vi "MTS_AutoZPos.vi"(0 "PH Dev":i32, 1 "OFlow Interv [s]":dbl, 2 "Accum Time [s]":dbl=0.1, 5 "PI System no.":i32, 11 "error in":errorcluster, 12 "Start Point":T1, 13 "Steps":i32=9, 14 "Step Width [um]":dbl=0.5) -> (4 "New Z":dbl, 6 "Counts":u32[](array[numeric]), 8 "Position":dbl[](array[numeric]), 15 "error out":errorcluster)   [LabVIEW 2013]
panel:
  out "FiFo Overrun":bool
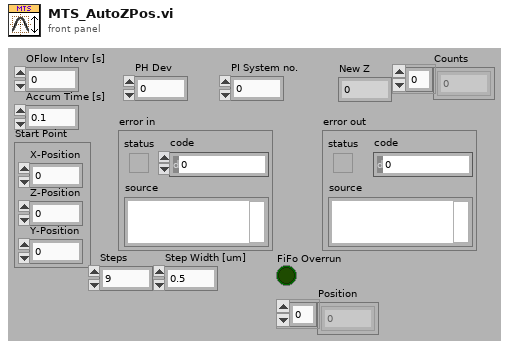
[diagram p1: front panel]
types:
  T1 = cluster{"X-Position":dbl, "Y-Position":dbl, "Z-Position":dbl}
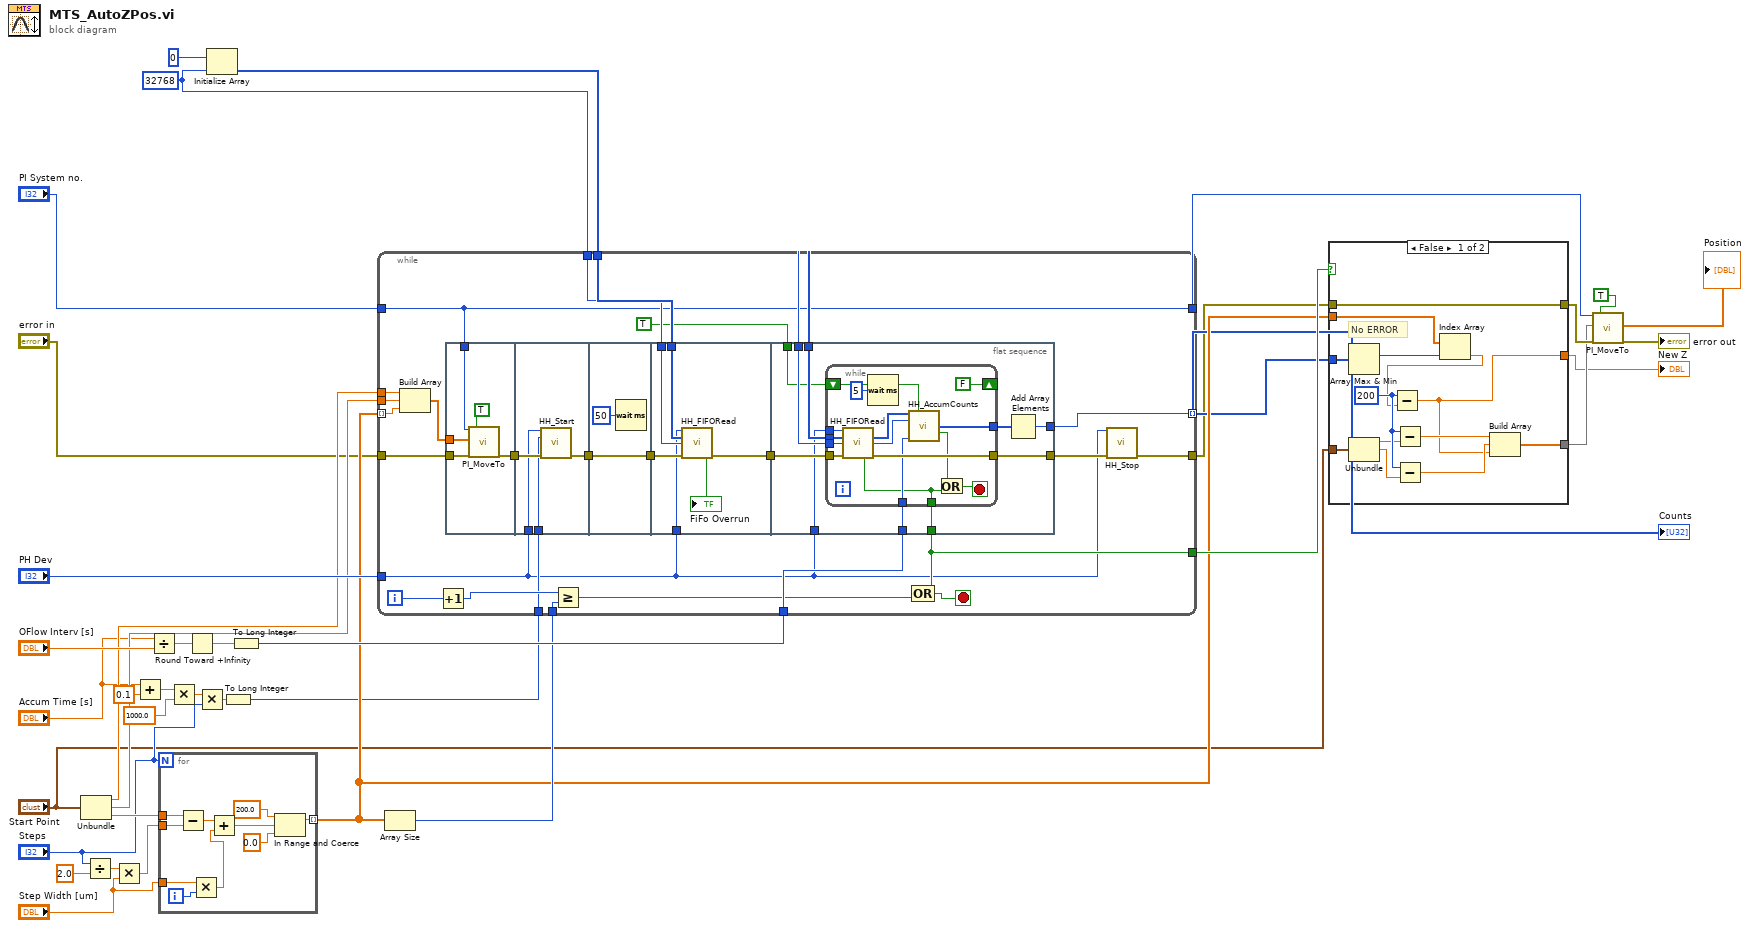
[diagram p0: block diagram]
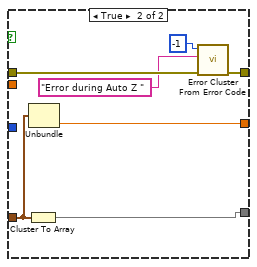
[diagram p2: hidden frame]
diagram:
  w2 = 32768 ("dimension size")
  n1 = Unbundle("Start Point") -> ("X-Position"=w23:dbl, "Y-Position"=w24:dbl, "Z-Position"=w27:dbl)
  n2 = Divide(x="Steps", y=2.0) -> (x/y=w30:dbl)
  n3 = Multiply(x=w30, y="Step Width [um]") -> (x*y=w26:dbl)
  n4 = Add(x="Accum Time [s]", y=0.1) -> (x+y=w19:dbl)
  n5 = Divide(x="Accum Time [s]", y="OFlow Interv [s]") -> (x/y=w33:dbl)
  n6 = for {
    N: "Steps" -> [_]
    tunnel: "Step Width [um]" -> [w47]
    tunnel: w27 -> [w46]
    tunnel: w26 -> [w43]
    tunnel: [w39] -> w10 mode=indexing
    i -> [w48]
    n7 = Subtract(x=w46, y=w43) -> (x-y=w42:dbl)
    n8 = Multiply(x=w47, y=w48) -> (x*y=w41:dbl)
    n9 = Add(x=w42, y=w41) -> (x+y=w40:dbl)
    n10 = In Range and Coerce(upper limit=200.0, x=w40, lower limit=0.0) -> (coerced(x)=w39:dbl)  [unwired: 1 out]
  }
  n11 = Multiply(x=w19, y=1000.0) -> (x*y=w17:dbl)
  n12 = Round Toward +Infinity(x=w33) -> (ceil(x): smallest int >= x=w32:dbl)
  n13 = Multiply(x=w17, y="Steps") -> (x*y=w15:dbl)
  n14 = Initialize Array(u32 0, w2) -> (w37:u32[])
  n15 = To Long Integer(number=w15) -> (32bit integer=w4:i32)
  n16 = To Long Integer(number=w32) -> (32bit integer=w31:i32)
  n17 = Array Size(array=w10) -> (size(s)=w25:i32)
  n18 = while {
    tunnel: "error in" -> [w71]
    tunnel: w37 -> [w70]
    tunnel: w2 -> [w69]
    tunnel: "PH Dev" -> [w49]
    tunnel: [w50] -> w3
    tunnel: "PI System no." -> [w56]
    tunnel: w31 -> [w67]
    tunnel: w25 -> [w64]
    tunnel: w10 -> [w59] mode=indexing
    tunnel: w24 -> [w60]
    tunnel: w23 -> [w61]
    tunnel: [w57] -> w22
    tunnel: [w56] -> w12
    tunnel: [w55] -> w6 mode=indexing
    tunnel: w4 -> [w52]
    i -> [w66]
    stop <- w63 stop-if-true
    n19 = Build Array(w61, w60, w59) -> (w58:dbl[])
    n20 = Increment(x=w66) -> (x+1=w65:i32)
    n21 = flat-sequence {
      tunnel: w71 -> [w78]
      tunnel: [w77] -> w54
      tunnel: w56 -> [w76]
      tunnel: w58 -> [w75]
      tunnel: w54 -> [w82]
      tunnel: [w81] -> w53
      tunnel: w52 -> [w80]
      tunnel: w49 -> [w79]
      tunnel: [w83] -> w73
      tunnel: w53 -> [w83]
      tunnel: w73 -> [w90]
      tunnel: w70 -> [w89]
      tunnel: w69 -> [w88]
      tunnel: w49 -> [w87]
      tunnel: [w86] -> w72
      tunnel: w70 -> [w99]
      tunnel: w69 -> [w98]
      tunnel: w49 -> [w97]
      tunnel: [w96] -> w51
      tunnel: w72 -> [w100]
      tunnel: TRUE ("Reset") -> [w95]
      tunnel: w67 -> [w93]
      tunnel: [w92] -> w55
      tunnel: [w91] -> w57
      frame #0 {
        n22 = call "PI_MoveTo.vi"("System no."=w76, "Target position"=w75, "error in"=w78, "Move"=TRUE) -> ("error out"=w77:errorcluster)  [unwired: 13 in, 2 out]
      }
      frame #1 {
        n23 = call "HH_Start.vi"("Device Index"=w79, "Acq. Time"=w80, "error in (no error)"=w82) -> ("error out"=w81:errorcluster)  [unwired: 11 in, 1 out]
      }
      frame #2 {
        n24 = Wait (ms)(milliseconds to wait=u32 50) -> ()  [unwired: 1 out]
      }
      frame #3 {
        n25 = call "HH_FIFORead.vi"("Device Index"=w87, "Buffer In"=w89, "Count"=w88, "error in (no error)"=w90) -> ("FiFo Overrun"=→"FiFo Overrun":bool, "error out"=w86:errorcluster)  [unwired: 7 in, 3 out]
      }
      frame #4 {
        n26 = while {
          tunnel: w100 -> [w115]
          tunnel: w99 -> [w114]
          tunnel: w98 -> [w113]
          tunnel: w97 -> [w112]
          tunnel: [w111] -> w96
          shift-right: [FALSE ("Reset")] -> _
          shift-left: w95 -> [w107]
          tunnel: [w105] -> w94
          tunnel: w93 -> [w104]
          tunnel: [w101] -> w91
          stop <- w102 stop-if-true
          n27 = call "HH_FIFORead.vi"("Device Index"=w112, "Buffer In"=w114, "Count"=w113, "error in (no error)"=w115) -> ("Buffer Out"=w109:u32[], "Data Count"=w110:i32, "FiFo Overrun"=w101:bool, "error out"=w111:errorcluster)  [unwired: 7 in, 1 out]
          n28 = Wait (ms)(milliseconds to wait=u32 5) -> ()  [unwired: 1 out]
          n29 = call "HH_AccumCounts.vi"("Data In"=w109, "Reset"=w107, "Data Count"=w110, "Acc X Overflows"=w104) -> ("Accum Counts"=w105:u32[], "Acc Time Ok"=w103:bool)  [unwired: 7 in, 3 out]
          n30 = Or(x=w103, y=w101) -> (x .or. y?=w102:bool)
        }
        n31 = Add Array Elements(numeric array=w94) -> (sum=w92:u32)
      }
    }
    n32 = Greater Or Equal?(x=w65, y=w64) -> (x >= y?=w62:bool)
    n33 = Compound Arithmetic op=OR(w57, w62) -> (w63:bool)
    n34 = call "HH_Stop.vi"("Device Index"=w49, "error in (no error)"=w51) -> ("error out"=w50:errorcluster)  [unwired: 12 in, 1 out]
  }
  "Counts" <- w6
  n35 = case shown="False" w22 {
    tunnel: w3 -> [w128 w135]
    tunnel: [w128 w134] -> w14
    tunnel: w6 -> [w127 _]
    tunnel: w10 -> [w126 _]
    tunnel: "Start Point" -> [w124 w130]
    tunnel: [w123 w131] -> w8
    tunnel: [w116 w129] -> w7
    frame False {
      w122 = 200
      # "No ERROR"
      n36 = Array Max & Min(array=w127) -> (max index (indices)=w125:i32)  [unwired: 3 out]
      n37 = Unbundle(w124) -> ("X-Position"=w121:dbl, "Y-Position"=w119:dbl)  [unwired: 1 out]
      n38 = Subtract(x=w122, y=w121) -> (x-y=w120:dbl)
      n39 = Subtract(x=w122, y=w119) -> (x-y=w118:dbl)
      n40 = Index Array(array=w126, index=w125) -> (element=w117:dbl)
      n41 = Subtract(x=w122, y=w117) -> (x-y=w116:dbl)
      n42 = Build Array(w120, w118, w116) -> (w123:dbl[])
    }
    frame True {
      n43 = Cluster To Array(cluster=w130) -> (array=w131:dbl[])
      n44 = Unbundle(w130) -> ("Z-Position"=w129:dbl)  [unwired: 2 out]
      n45 = call <vilib>:"Error Cluster From Error Code.vi"("error in (no error)"=w135, "error message (\"\")"="Error during Auto Z " ("error message (\"\")"), "error code (0)"=-1) -> ("error out"=w134:errorcluster)  [unwired: 6 in]
    }
  }
  "New Z" <- w7
  n46 = call "PI_MoveTo.vi"("System no."=w12, "Target position"=w8, "error in"=w14, "Move"=TRUE) -> ("Position"=→"Position":dbl[], "error out"=→"error out":errorcluster)  [unwired: 13 in, 1 out]
